vi "Save Color Range to NT Tables.vi"(8 "error in":errorcluster, 9 "Color Range":T1={"Hue"={103, 151}, "Sat"={217, 255}, "Val"={201, 249}} {"Val" scale format="%#.0f"; "Sat" scale format="%#.0f"; "Hue" scale=0.0..255.0 scale format="%#.0f"}, 11 "Color Range Name":string="/Vision/BallColorRange") -> (0 "error out":errorcluster, 2 "appended array":u8[](array[numeric]))   [LabVIEW 2025]
uses:
  <vilib>/Rock Robotics/Network Tables/NT Write Integer Array.vi
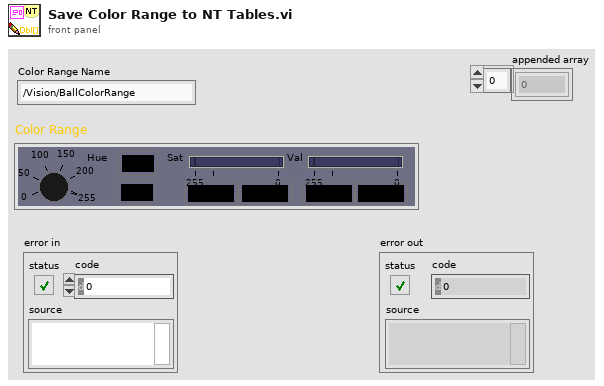
[diagram p1: front panel]
types:
  T1 = cluster{"Hue":cluster{i64, i64}, "Sat":cluster{i64, i64}, "Val":cluster{i64, i64}}
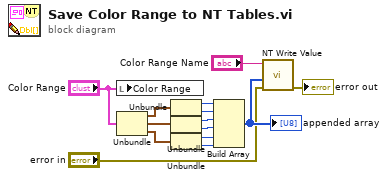
[diagram p0: block diagram]
diagram:
  n1 = local write "Color Range"("Color Range") -> ()
  n2 = Unbundle("Color Range") -> ("Hue"=w3:cluster{i64, i64}, "Sat"=w2:cluster{i64, i64}, "Val"=w1:cluster{i64, i64})
  n3 = Unbundle(w3) -> (w14:i64, w13:i64)
  n4 = Unbundle(w2) -> (w11:i64, w12:i64)
  n5 = Unbundle(w1) -> (w10:i64, w9:i64)
  n6 = Build Array(w14, w13, w11, w12, w10, w9) -> (w8:i64[])
  "appended array" <- w8
  n7 = call-poly <vilib>:"NT Write Value.vi"("error in"="error in", "value"=w8, "name"="Color Range Name") -> ("error out"=→"error out":errorcluster)  [unwired: 8 in]
